vi "Write Multi Single.vi"(0 "Device ID":T4(ring), 2 "Output_Action":enum8{"Off", "On"}[](array[ring]), 5 "Module":T3(array[ring]), 7 "Single_Output":T2(array[ring]), 9 "Output_PWM":T1(array[ring]), 11 "error in":errorcluster) -> (4 "Device ID Out":T4(ring), 15 "error out":errorcluster)   [LabVIEW 2010]
doc: "This VI writes multiple single-ended digital PWM output signals to the transfer area."
uses:
  Robo Interface.dll
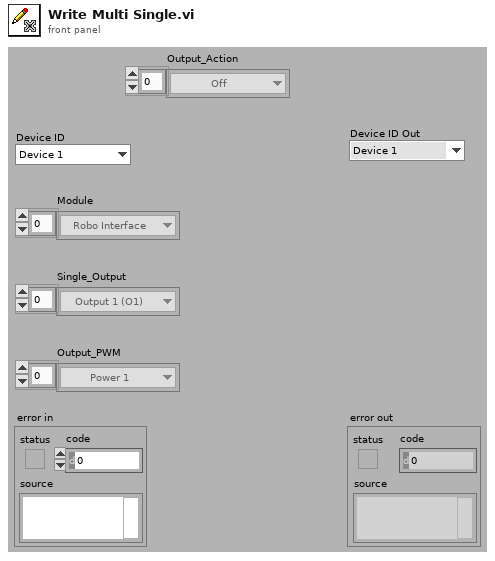
[diagram p1: front panel]
types:
  T1 = enum8{"Power 1", "Power 2", "Power 3", "Power 4", "Power 5", "Power 6", "Power 7", "Power 8"}[]
  T2 = enum8{"Output 1 (O1)", "Output 2 (O2)", "Output 3 (O3)", "Output 4 (O4)", "Output 5 (O5)", "Output 6 (O6)", "Output 7 (O7)", "Output 8 (O8)"}[]
  T3 = enum8{"Robo Interface", "Extension 1", "Extension 2", "Extension 3"}[]
  T4 = enum16{"Device 1", "Device 2", "Device 3", "Device 4", "Device 5", "Device 6", "Device 7", "Device 8"}
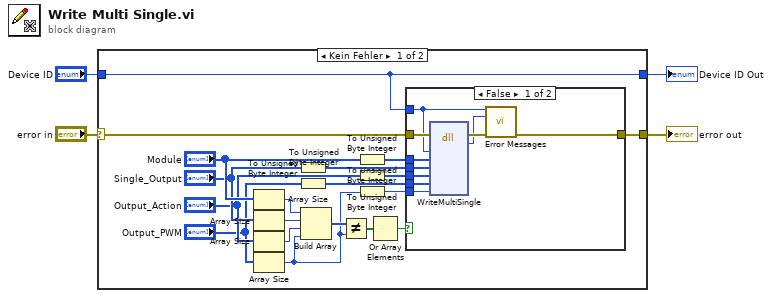
[diagram p0: block diagram]
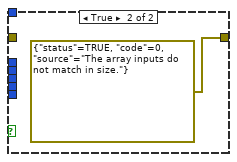
[diagram p2: hidden frame]
diagram:
  n1 = case shown="Kein Fehler" "error in" {
    selector: "error in" -> [w23 w36]
    tunnel: [w22 w36] -> w1
    tunnel: "Device ID" -> [w5 w35]
    tunnel: [w5 w35] -> w2
    frame No Error {
      n2 = Array Size(array="Module") -> (size(s)=w21:i32)
      n3 = Array Size(array="Single_Output") -> (size(s)=w20:i32)
      n4 = Array Size(array="Output_Action") -> (size(s)=w19:i32)
      n5 = Array Size(array="Output_PWM") -> (size(s)=w16:i32)
      n6 = To Unsigned Byte Integer(number="Single_Output") -> (unsigned 8bit integer=w10:u8[])
      n7 = To Unsigned Byte Integer(number="Output_PWM") -> (unsigned 8bit integer=w8:u8[])
      n8 = Build Array(w21, w20, w19, w16) -> (w18:i32[])
      n9 = Not Equal?(x=w18, y=w16) -> (x != y?=w17:bool[])
      n10 = To Unsigned Byte Integer(number="Module") -> (unsigned 8bit integer=w11:u8[])
      n11 = To Unsigned Byte Integer(number="Output_Action") -> (unsigned 8bit integer=w9:u8[])
      n12 = To Unsigned Byte Integer(number=w16) -> (unsigned 8bit integer=w13:u8)
      n13 = Or Array Elements(Boolean array=w17) -> (logical OR=w12:bool)
      n14 = case shown="FALSE" w12 {
        tunnel: w23 -> [w33 _]
        tunnel: [w31 errorcluster {"status"=TRUE, "code"=0, "source"="The array inputs do not match in size."} ("error out")] -> w22
        tunnel: w11 -> [w26 _]
        tunnel: w10 -> [w27 _]
        tunnel: w9 -> [w28 _]
        tunnel: w8 -> [w29 _]
        tunnel: w13 -> [w30 _]
        tunnel: w5 -> [w24 _]
        frame False {
          n15 = dll-call lib="D:/Aron/LabVIEW-Programmierung/a.F.b.u.s.A/robo_interface_distribute/Robo Interface/Advanced/Robo Interface.dll" fn="WriteMultiSingle"(error in=w33, "Device_ID"=w24, "Module"=w26, "Single_Output"=w27, "Output_Action"=w28, "Output_PWM"=w29, "Array_Legnth"=w30) -> (error out=w32:errorcluster, "return type"=w25:i32)  [unwired: 7 in, 2 out]
          n16 = call "Error Messages.vi"("Device ID"=w24, "Error Code"=w25, "error in (no error)"=w32) -> ("error out"=w31:errorcluster)  [unwired: 12 out]
        }
        frame True {
        }
      }
    }
    frame Error {
    }
  }
  "error out" <- w1
  "Device ID Out" <- w2
